vi "Range Kontrol X.vi"(0 "denge degeri":dbl, 1 "iterasyon Denge":dbl=1.0, 2 "frekans index":dbl, 3 "Denge Kosulu x1_x2":dbl[][](array[numeric]), 4 "Xk":dbl, 5 "X(k-1)":dbl=0.1, 6 "output x 1":dbl, 7 "output x 2":dbl) -> (14 "Output X(k-1)":dbl format="%.4p", 15 "result output x":dbl, 17 "KONTROL Y":bool, 18 "IF ELSE":bool, 19 "Start Denge Y":bool)   [LabVIEW 2014]
uses:
  Sub_VI/show_sensitivity.vi
  Sub_VI/global get findinput.vi
panel:
  in  "GPIB In":refnum<visa-resource-name>="GPIB0::8::INSTR"
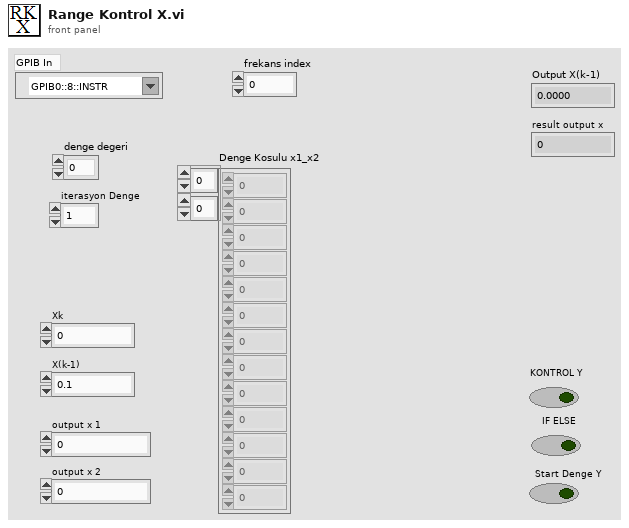
[diagram p1: front panel]
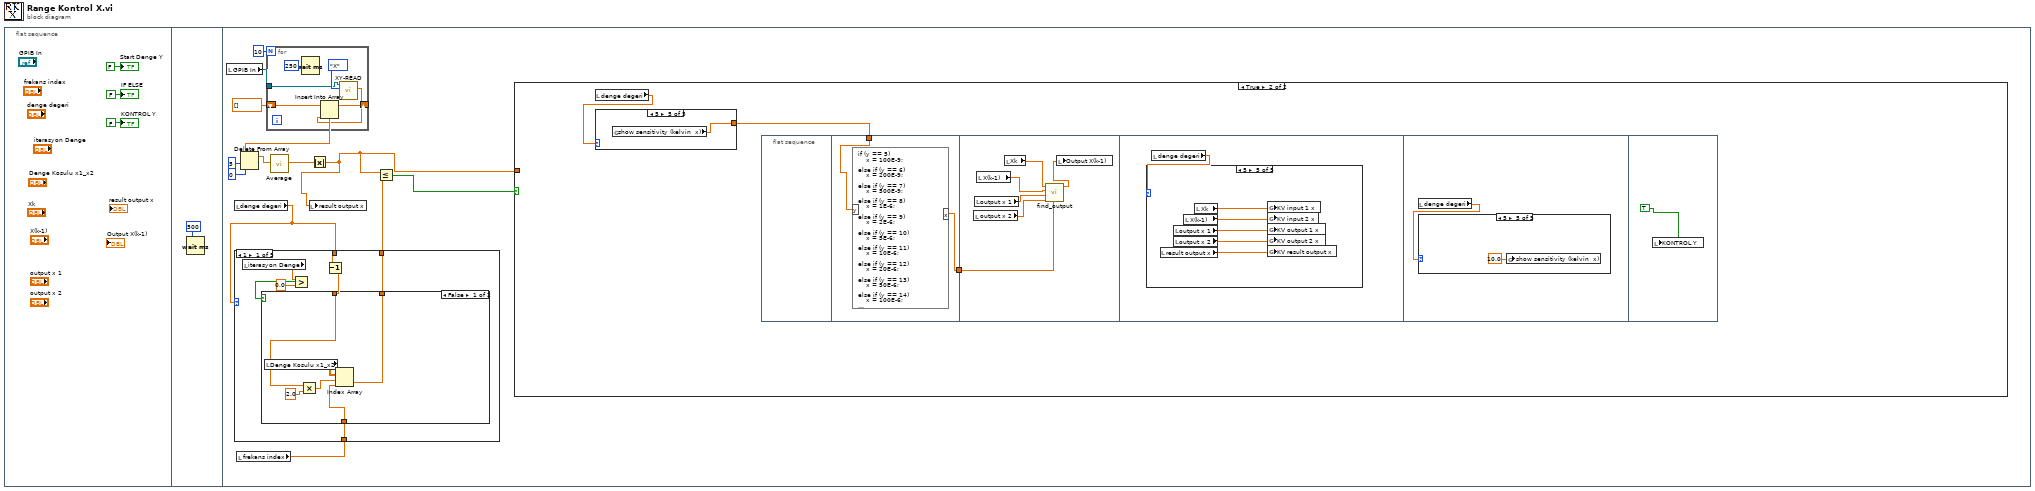
[diagram p0: block diagram]
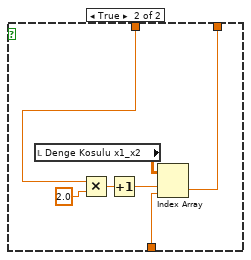
[diagram p2: hidden frame]
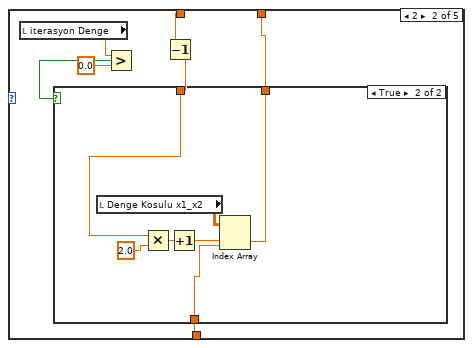
[diagram p3: hidden frame]
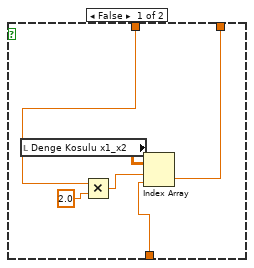
[diagram p4: hidden frame]
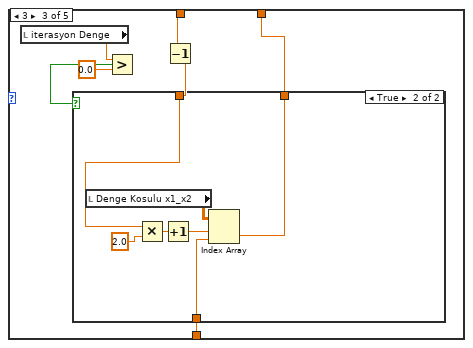
[diagram p5: hidden frame]
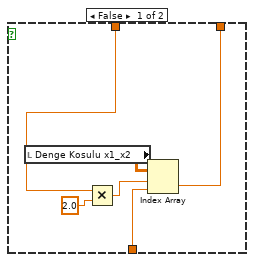
[diagram p6: hidden frame]
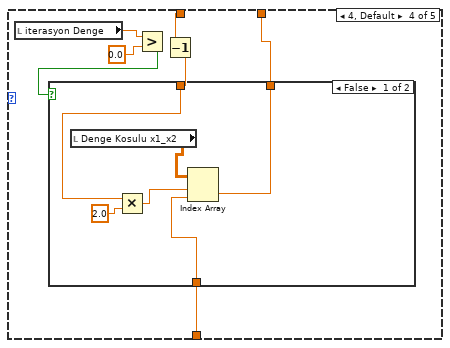
[diagram p7: hidden frame]
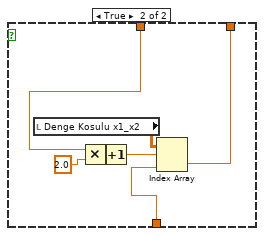
[diagram p8: hidden frame]
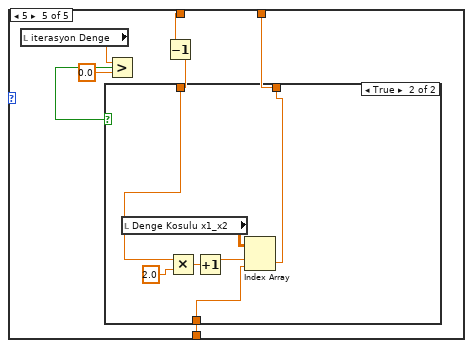
[diagram p9: hidden frame]
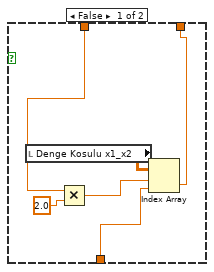
[diagram p10: hidden frame]
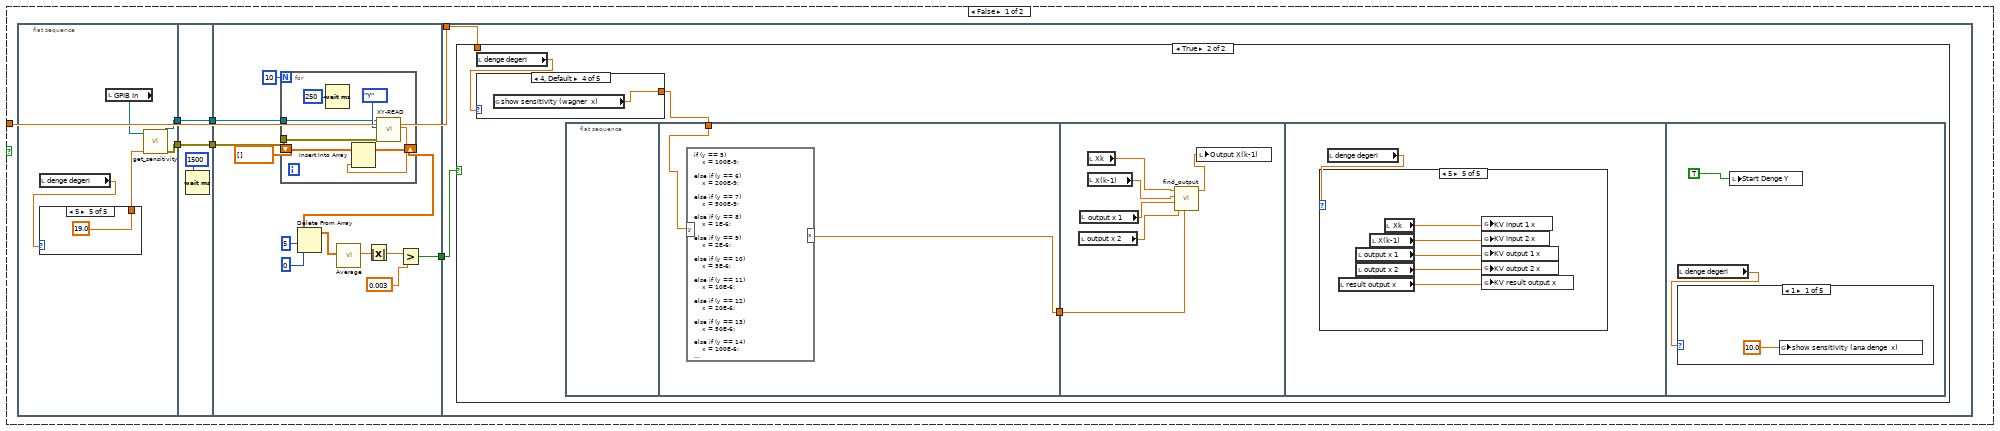
[diagram p11: hidden frame]
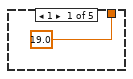
[diagram p12: hidden frame]
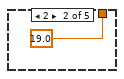
[diagram p13: hidden frame]
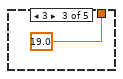
[diagram p14: hidden frame]
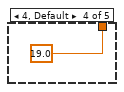
[diagram p15: hidden frame]
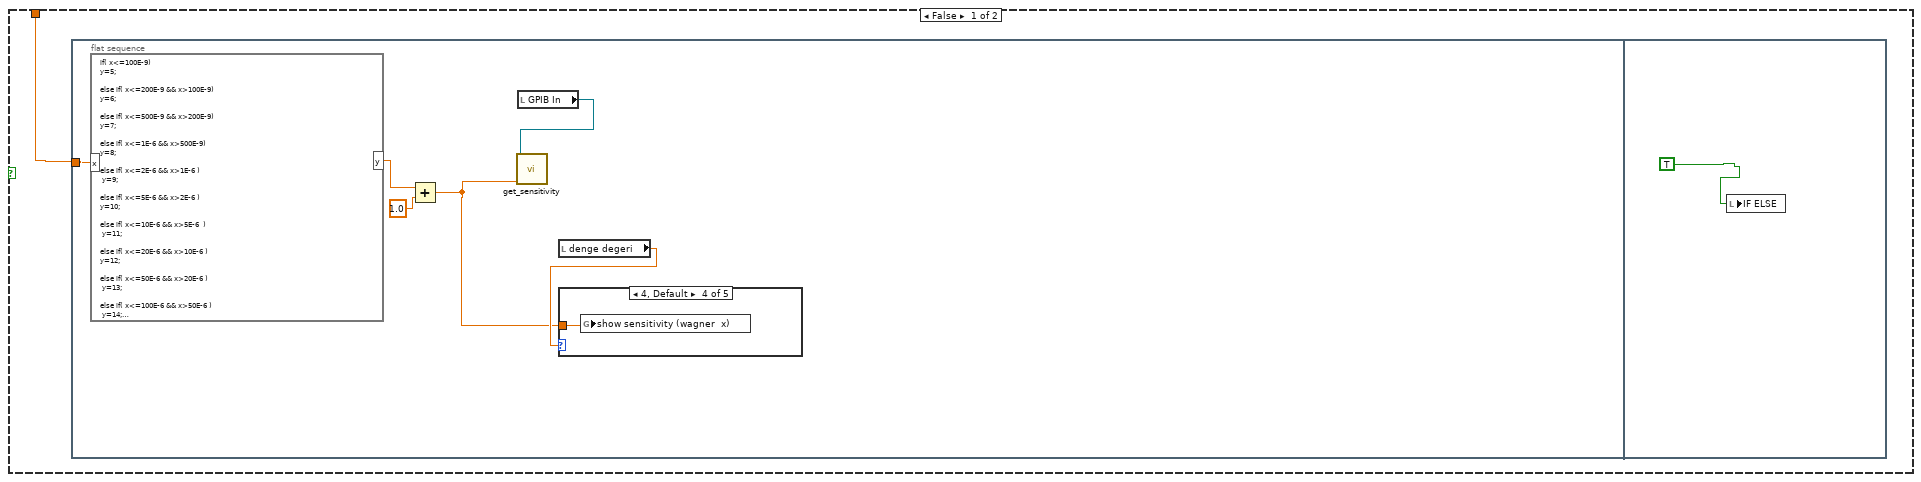
[diagram p16: hidden frame]
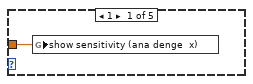
[diagram p17: hidden frame]
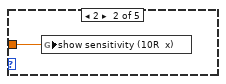
[diagram p18: hidden frame]
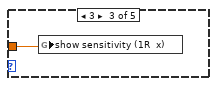
[diagram p19: hidden frame]
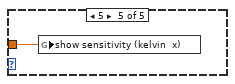
[diagram p20: hidden frame]
diagram:
  n1 = flat-sequence {
    frame #0 {
      "Start Denge Y" <- FALSE ("Denge Y")
      "IF ELSE" <- FALSE ("IF ELSE")
      "KONTROL Y" <- FALSE ("KONTROL Y")
    }
    frame #1 {
      n2 = Wait (ms)(milliseconds to wait=u32 500) -> ()  [unwired: 1 out]
    }
    frame #2 {
      n3 = local read "GPIB In"() -> (w5:refnum<visa-resource-name>)
      n4 = local read "denge degeri"() -> (w8:dbl)
      n5 = local read "frekans index"() -> (w6:dbl)
      n6 = case shown="1" w8 {
        tunnel: [w21 w41 w61 w84 w101] -> w9
        tunnel: w8 -> [w20 w40 w60 w80 w100]
        tunnel: w6 -> [w18 w38 w58 w78 w98]
        frame 1 {
          n7 = local read "iterasyon Denge"() -> (w23:dbl)
          n8 = Greater?(x=w23, y=0.0) -> (0:w24:bool)
          n9 = Decrement(x=w20) -> (x-1=w19:dbl)
          n10 = case shown="False" w24 {
            tunnel: [w28 w34] -> w21
            tunnel: w19 -> [w27 w33]
            tunnel: w18 -> [w25 w31]
            frame False {
              n11 = local read "Denge Kosulu x1_x2"() -> (w30:dbl[][])
              n12 = Multiply(x=w27, y=2.0) -> (x*y=w26:dbl)
              n13 = Index Array(array=w30, index (row)=w26, index (col)=w25) -> (element=w28:dbl)
            }
            frame True {
              n14 = local read "Denge Kosulu x1_x2"() -> (w35:dbl[][])
              n15 = Multiply(x=w33, y=2.0) -> (x*y=w37:dbl)
              n16 = Increment(x=w37) -> (x+1=w32:dbl)
              n17 = Index Array(array=w35, index (row)=w32, index (col)=w31) -> (element=w34:dbl)
            }
          }
        }
        frame 2 {
          n18 = local read "iterasyon Denge"() -> (w43:dbl)
          n19 = Greater?(x=w43, y=0.0) -> (0:w44:bool)
          n20 = Decrement(x=w40) -> (x-1=w39:dbl)
          n21 = case shown="True" w44 {
            tunnel: [w48 w54] -> w41
            tunnel: w39 -> [w47 w53]
            tunnel: w38 -> [w45 w51]
            frame False {
              n22 = local read "Denge Kosulu x1_x2"() -> (w50:dbl[][])
              n23 = Multiply(x=w47, y=2.0) -> (x*y=w46:dbl)
              n24 = Index Array(array=w50, index (row)=w46, index (col)=w45) -> (element=w48:dbl)
            }
            frame True {
              n25 = local read "Denge Kosulu x1_x2"() -> (w55:dbl[][])
              n26 = Multiply(x=w53, y=2.0) -> (x*y=w57:dbl)
              n27 = Increment(x=w57) -> (x+1=w52:dbl)
              n28 = Index Array(array=w55, index (row)=w52, index (col)=w51) -> (element=w54:dbl)
            }
          }
        }
        frame 3 {
          n29 = local read "iterasyon Denge"() -> (w62:dbl)
          n30 = Greater?(x=w62, y=0.0) -> (0:w64:bool)
          n31 = Decrement(x=w60) -> (x-1=w59:dbl)
          n32 = case shown="True" w64 {
            tunnel: [w68 w74] -> w61
            tunnel: w59 -> [w67 w73]
            tunnel: w58 -> [w65 w71]
            frame False {
              n33 = local read "Denge Kosulu x1_x2"() -> (w70:dbl[][])
              n34 = Multiply(x=w67, y=2.0) -> (x*y=w66:dbl)
              n35 = Index Array(array=w70, index (row)=w66, index (col)=w65) -> (element=w68:dbl)
            }
            frame True {
              n36 = local read "Denge Kosulu x1_x2"() -> (w75:dbl[][])
              n37 = Multiply(x=w73, y=2.0) -> (x*y=w77:dbl)
              n38 = Increment(x=w77) -> (x+1=w72:dbl)
              n39 = Index Array(array=w75, index (row)=w72, index (col)=w71) -> (element=w74:dbl)
            }
          }
        }
        frame 4, Default {
          n40 = local read "iterasyon Denge"() -> (w82:dbl)
          n41 = Greater?(x=w82, y=0.0) -> (0:w81:bool)
          n42 = Decrement(x=w80) -> (x-1=w79:dbl)
          n43 = case shown="False" w81 {
            tunnel: [w88 w94] -> w84
            tunnel: w79 -> [w87 w93]
            tunnel: w78 -> [w85 w91]
            frame False {
              n44 = local read "Denge Kosulu x1_x2"() -> (w90:dbl[][])
              n45 = Multiply(x=w87, y=2.0) -> (x*y=w86:dbl)
              n46 = Index Array(array=w90, index (row)=w86, index (col)=w85) -> (element=w88:dbl)
            }
            frame True {
              n47 = local read "Denge Kosulu x1_x2"() -> (w95:dbl[][])
              n48 = Multiply(x=w93, y=2.0) -> (x*y=w97:dbl)
              n49 = Increment(x=w97) -> (x+1=w92:dbl)
              n50 = Index Array(array=w95, index (row)=w92, index (col)=w91) -> (element=w94:dbl)
            }
          }
        }
        frame 5 {
          n51 = local read "iterasyon Denge"() -> (w102:dbl)
          n52 = Greater?(x=w102, y=0.0) -> (0:w104:bool)
          n53 = Decrement(x=w100) -> (x-1=w99:dbl)
          n54 = case shown="True" w104 {
            tunnel: [w108 w114] -> w101
            tunnel: w99 -> [w107 w113]
            tunnel: w98 -> [w105 w111]
            frame False {
              n55 = local read "Denge Kosulu x1_x2"() -> (w110:dbl[][])
              n56 = Multiply(x=w107, y=2.0) -> (x*y=w106:dbl)
              n57 = Index Array(array=w110, index (row)=w106, index (col)=w105) -> (element=w108:dbl)
            }
            frame True {
              n58 = local read "Denge Kosulu x1_x2"() -> (w115:dbl[][])
              n59 = Multiply(x=w113, y=2.0) -> (x*y=w117:dbl)
              n60 = Increment(x=w117) -> (x+1=w112:dbl)
              n61 = Index Array(array=w115, index (row)=w112, index (col)=w111) -> (element=w114:dbl)
            }
          }
        }
      }
      n62 = for {
        N: 10 -> [_]
        shift-right: [w271] -> w14
        shift-left: dbl[] [] -> [w272]
        tunnel: w5 -> [w269]
        n63 = Wait (ms)(milliseconds to wait=u32 250) -> ()  [unwired: 1 out]
        n64 = call "XY-READ.vi"("X/Y ?"=enum16{"X", "Y"}."X" ("Enum"), "SR850 GPIB IN"=w269) -> ("SR850_Reading"=w273:dbl)  [unwired: 7 in, 2 out]
        n65 = Insert Into Array(array=w272, new element=w273) -> (w271:dbl[])  [unwired: 1 in]
      }
      n66 = Delete From Array(array=w14, length=5, index=0) -> (array with subset deleted=w15:dbl[])  [unwired: 1 out]
      n67 = call "Average.vi"("Array"=w15) -> ("Average"=w11:dbl)  [unwired: 9 in, 1 out]
      n68 = Absolute Value(x=w11) -> (abs(x)=w7:dbl)
      n69 = local write "result output x"(w7) -> ()
      n70 = Less Or Equal?(x=w7, y=w9) -> (x <= y?=w10:bool)
      n71 = case shown="True" w10 {
        tunnel: w7 -> [w118 _]
        frame False {
          n72 = flat-sequence {
            tunnel: [w127] -> w122
            tunnel: [w126] -> w120
            tunnel: [w135] -> w123
            tunnel: w122 -> [w135]
            tunnel: [w134] -> w121
            tunnel: w120 -> [w134]
            tunnel: w123 -> [w142]
            tunnel: w121 -> [w141]
            tunnel: [w138] -> w119
            tunnel: w119 -> [w157]
            tunnel: w118 -> [w156]
            frame #0 {
              n73 = local read "denge degeri"() -> (w125:dbl)
              n74 = case shown="5" w125 {
                tunnel: [19.0 ("input 1") 19.0 ("input 1") 19.0 ("input 1") 19.0 ("input 1") 19.0 ("input 1")] -> w124
                frame 1 {
                }
                frame 2 {
                }
                frame 3 {
                }
                frame 4, Default {
                }
                frame 5 {
                }
              }
              n75 = local read "GPIB In"() -> (w128:refnum<visa-resource-name>)
              n76 = call "get_sensitivity.vi"("input 1"=w124, "SR850 GPIB In"=w128) -> ("error out"=w126:errorcluster, "SR850 GPIB Out"=w127:refnum<visa-resource-name>)  [unwired: 8 in]
            }
            frame #1 {
              n77 = Wait (ms)(milliseconds to wait=u32 1500) -> ()  [unwired: 1 out]
            }
            frame #2 {
              n78 = for {
                N: 10 -> [_]
                tunnel: w142 -> [w154]
                tunnel: w141 -> [w153]
                shift-right: [w150] -> w146
                shift-left: dbl[] [] -> [w151]
                n79 = Wait (ms)(milliseconds to wait=u32 250) -> ()  [unwired: 1 out]
                n80 = call "XY-READ.vi"("Error IN"=w153, "X/Y ?"=enum16{"X", "Y"}."Y" ("Enum"), "SR850 GPIB IN"=w154) -> ("SR850_Reading"=w152:dbl)  [unwired: 6 in, 2 out]
                n81 = Insert Into Array(array=w151, new element=w152) -> (w150:dbl[])  [unwired: 1 in]
              }
              n82 = Delete From Array(array=w146, length=5, index=0) -> (array with subset deleted=w145:dbl[])  [unwired: 1 out]
              n83 = call "Average.vi"("Array"=w145) -> ("Average"=w139:dbl)  [unwired: 9 in, 1 out]
              n84 = Absolute Value(x=w139) -> (abs(x)=w137:dbl)
              n85 = Greater?(x=w137, y=0.003) -> (0:w138:bool)
            }
            frame #3 {
              n86 = case shown="True" w157 {
                tunnel: w156 -> [w158 _]
                frame False {
                  n87 = flat-sequence {
                    tunnel: w158 -> [w163]
                    frame #0 {
                      n88 = formula code="if( x<=100E-9) \ny=5;\n\nelse if( x<=200E-9 && x>100E-9) \ny=6;\n\nelse if( x<=500E-9 && x>200E-9) \ny=7;\n\nelse if( x<=1E-6 && x>500E-9) \ny=8;\n\nelse if( x<=2E-6 && x>1E-6 ) \n\ty=9;\n\nelse if( x<=5E-6 && x>2E-6 ) \ny=10;\n\nelse if( x<=10E-6 && x>5E-6  ) \n\ty=11;\n\nelse if( x<=20E-6 && x>10E-6 ) \ny=12;\n\nelse if( x<=50E-6 && x>20E-6 ) \n\ty=13;\n\nelse if( x<=100E-6 && x>50E-6 ) \n\ty=14;\n\nelse if( x<=200E-6 && x>100E-6 ) \n\ty=15;\n\nelse if( x<=500E-6 && x>200E-6 ) \n\ty=16;\n\nelse if(  x<=1E-3 && x>500E-6 ) \n\ty=17;\n\nelse if( x<=2E-3 && x>1E-3 ) \n\ty=18;\n\nelse if(  x<=5E-3 && x>2E-3) \ny=19;\n\nelse if(  x<=10E-3 && x>5E-3 ) \n\ty=20;\n\nelse if(  x<=20E-3 && x>10E-3) \n\ty=21;\n\nelse if(  x<=50E-3 && x>20E-3 ) \n\ty=22;\n\nelse if(  x<=100E-3 && x>50E-3 ) \n\ty=23;\n\nelse if(  x<=200E-3 && x>100E-3 ) \n\ty=24;\n\nelse if(  x<=500E-3 && x>200E-3 ) \n\ty=25;\n\nelse if(  x<=1 && x>500E-3 ) \ny=26;\n\nelse \n\ty=26;"("x"=w163) -> ("y"=w161:dbl)
                      n89 = Add(x=w161, y=1.0) -> (x+y=w159:dbl)
                      n90 = local read "GPIB In"() -> (w164:refnum<visa-resource-name>)
                      n91 = call "get_sensitivity.vi"("input 1"=w159, "SR850 GPIB In"=w164) -> ()  [unwired: 8 in, 2 out]
                      n92 = local read "denge degeri"() -> (w162:dbl)
                      n93 = case shown="4, Default" w162 {
                        tunnel: w159 -> [w165 w166 w167 w168 w169]
                        frame 1 {
                          n94 = global write "show_sensitivity.vi" "show sensitivity (ana denge  x)"(w165) -> ()
                        }
                        frame 2 {
                          n95 = global write "show_sensitivity.vi" "show sensitivity (10R  x)"(w166) -> ()
                        }
                        frame 3 {
                          n96 = global write "show_sensitivity.vi" "show sensitivity (1R  x)"(w167) -> ()
                        }
                        frame 4, Default {
                          n97 = global write "show_sensitivity.vi" "show sensitivity (wagner  x)"(w168) -> ()
                        }
                        frame 5 {
                          n98 = global write "show_sensitivity.vi" "show sensitivity (kelvin  x)"(w169) -> ()
                        }
                      }
                    }
                    frame #1 {
                      n99 = local write "IF ELSE"(TRUE ("if else")) -> ()
                    }
                  }
                }
                frame True {
                  n100 = local read "denge degeri"() -> (w172:dbl)
                  n101 = case shown="4, Default" w172 {
                    tunnel: [w174 w175 w176 w177 w178] -> w171
                    frame 1 {
                      n102 = global read "show_sensitivity.vi" "show sensitivity (ana denge  x)"() -> (w174:dbl)
                    }
                    frame 2 {
                      n103 = global read "show_sensitivity.vi" "show sensitivity (10R  x)"() -> (w175:dbl)
                    }
                    frame 3 {
                      n104 = global read "show_sensitivity.vi" "show sensitivity (1R  x)"() -> (w176:dbl)
                    }
                    frame 4, Default {
                      n105 = global read "show_sensitivity.vi" "show sensitivity (wagner  x)"() -> (w177:dbl)
                    }
                    frame 5 {
                      n106 = global read "show_sensitivity.vi" "show sensitivity (kelvin  x)"() -> (w178:dbl)
                    }
                  }
                  n107 = flat-sequence {
                    tunnel: w171 -> [w179]
                    tunnel: [w180] -> w173
                    tunnel: w173 -> [w184]
                    frame #0 {
                    }
                    frame #1 {
                      n108 = formula code="if (y == 5) \n    x = 100E-9;\n\nelse if (y == 6) \n    x = 200E-9;\n\nelse if (y == 7) \n    x = 500E-9;\n\nelse if (y == 8) \n    x = 1E-6;\n\nelse if (y == 9) \n    x = 2E-6;\n\nelse if (y == 10) \n    x = 5E-6;\n\nelse if (y == 11) \n    x = 10E-6;\n\nelse if (y == 12) \n    x = 20E-6;\n\nelse if (y == 13) \n    x = 50E-6;\n\nelse if (y == 14) \n    x = 100E-6;\n\nelse if (y == 15) \n    x = 200E-6;\n\nelse if (y == 16) \n    x = 500E-6;\n\nelse if (y == 17) \n    x = 1E-3;\n\nelse if (y == 18) \n    x = 2E-3;\n\nelse if (y == 19) \n    x = 5E-3;\n\nelse if (y == 20) \n    x = 10E-3;\n\nelse if (y == 21) \n    x = 20E-3;\n\nelse if (y == 22) \n    x = 50E-3;\n\nelse if (y == 23) \n    x = 100E-3;\n\nelse if (y == 24) \n    x = 200E-3;\n\nelse if (y == 25) \n    x = 500E-3;\n\nelse if (y == 26) \n    x = 1;\n\nelse \n    x = 1;"("y"=w179) -> ("x"=w180:dbl)
                    }
                    frame #2 {
                      n109 = local read "output x 2"() -> (w185:dbl)
                      n110 = local read "output x 1"() -> (w186:dbl)
                      n111 = local read "Xk"() -> (w181:dbl)
                      n112 = local read "X(k-1)"() -> (w182:dbl)
                      n113 = call "find_output.vi"("find output"=w184, "output 2"=w185, "output 1"=w186, "input 2"=w182, "input 1"=w181) -> ("getInput"=w183:dbl)  [unwired: 6 in]
                      n114 = local write "Output X(k-1)"(w183) -> ()
                    }
                    frame #3 {
                      n115 = local read "denge degeri"() -> (w187:dbl)
                      n116 = case shown="5" w187 {
                        frame 1 {
                          n117 = local read "result output x"() -> (w188:dbl)
                          n118 = local read "output x 1"() -> (w190:dbl)
                          n119 = local read "output x 2"() -> (w189:dbl)
                          n120 = local read "X(k-1)"() -> (w191:dbl)
                          n121 = local read "Xk"() -> (w192:dbl)
                          n122 = global write "global get findinput.vi" "AD input 1 x"(w192) -> ()
                          n123 = global write "global get findinput.vi" "AD input 2 x"(w191) -> ()
                          n124 = global write "global get findinput.vi" "AD output 1 x"(w190) -> ()
                          n125 = global write "global get findinput.vi" "AD output 2 x"(w189) -> ()
                          n126 = global write "global get findinput.vi" "AD result output x"(w188) -> ()
                        }
                        frame 2 {
                          n127 = local read "result output x"() -> (w193:dbl)
                          n128 = local read "output x 1"() -> (w195:dbl)
                          n129 = local read "output x 2"() -> (w194:dbl)
                          n130 = local read "X(k-1)"() -> (w196:dbl)
                          n131 = local read "Xk"() -> (w197:dbl)
                          n132 = global write "global get findinput.vi" "10R input 1 x"(w197) -> ()
                          n133 = global write "global get findinput.vi" "10R input 2 x"(w196) -> ()
                          n134 = global write "global get findinput.vi" "10R output 1 x"(w195) -> ()
                          n135 = global write "global get findinput.vi" "10R output 2 x"(w194) -> ()
                          n136 = global write "global get findinput.vi" "10R result output x"(w193) -> ()
                        }
                        frame 3 {
                          n137 = local read "result output x"() -> (w198:dbl)
                          n138 = local read "output x 1"() -> (w200:dbl)
                          n139 = local read "output x 2"() -> (w199:dbl)
                          n140 = local read "X(k-1)"() -> (w201:dbl)
                          n141 = local read "Xk"() -> (w202:dbl)
                          n142 = global write "global get findinput.vi" "1R input 1 x"(w202) -> ()
                          n143 = global write "global get findinput.vi" "1R input 2 x"(w201) -> ()
                          n144 = global write "global get findinput.vi" "1R output 1 x"(w200) -> ()
                          n145 = global write "global get findinput.vi" "1R output 2 x"(w199) -> ()
                          n146 = global write "global get findinput.vi" "1R result output x"(w198) -> ()
                        }
                        frame 4, Default {
                          n147 = local read "result output x"() -> (w203:dbl)
                          n148 = local read "output x 1"() -> (w205:dbl)
                          n149 = local read "output x 2"() -> (w204:dbl)
                          n150 = local read "X(k-1)"() -> (w206:dbl)
                          n151 = local read "Xk"() -> (w207:dbl)
                          n152 = global write "global get findinput.vi" "W input 1 x"(w207) -> ()
                          n153 = global write "global get findinput.vi" "W input 2 x"(w206) -> ()
                          n154 = global write "global get findinput.vi" "W output 1 x"(w205) -> ()
                          n155 = global write "global get findinput.vi" "W output 2 x"(w204) -> ()
                          n156 = global write "global get findinput.vi" "W result output x"(w203) -> ()
                        }
                        frame 5 {
                          n157 = local read "result output x"() -> (w208:dbl)
                          n158 = local read "output x 1"() -> (w209:dbl)
                          n159 = local read "output x 2"() -> (w210:dbl)
                          n160 = local read "X(k-1)"() -> (w211:dbl)
                          n161 = local read "Xk"() -> (w212:dbl)
                          n162 = global write "global get findinput.vi" "KV input 1 x"(w212) -> ()
                          n163 = global write "global get findinput.vi" "KV input 2 x"(w211) -> ()
                          n164 = global write "global get findinput.vi" "KV output 1 x"(w209) -> ()
                          n165 = global write "global get findinput.vi" "KV output 2 x"(w210) -> ()
                          n166 = global write "global get findinput.vi" "KV result output x"(w208) -> ()
                        }
                      }
                    }
                    frame #4 {
                      n167 = local read "denge degeri"() -> (w213:dbl)
                      n168 = case shown="1" w213 {
                        frame 1 {
                          n169 = global write "show_sensitivity.vi" "show sensitivity (ana denge  x)"(10.0 ("show sensitivity (kelvin  x)")) -> ()
                        }
                        frame 2 {
                          n170 = global write "show_sensitivity.vi" "show sensitivity (10R  x)"(16.0 ("show sensitivity (kelvin  x)")) -> ()
                        }
                        frame 3 {
                          n171 = global write "show_sensitivity.vi" "show sensitivity (1R  x)"(16.0 ("show sensitivity (kelvin  x)")) -> ()
                        }
                        frame 4, Default {
                          n172 = global write "show_sensitivity.vi" "show sensitivity (wagner  x)"(16.0 ("show sensitivity (kelvin  x)")) -> ()
                        }
                        frame 5 {
                          n173 = global write "show_sensitivity.vi" "show sensitivity (kelvin  x)"(10.0 ("show sensitivity (kelvin  x)")) -> ()
                        }
                      }
                      n174 = local write "Start Denge Y"(TRUE ("WAGNER Y")) -> ()
                    }
                  }
                }
              }
            }
          }
        }
        frame True {
          n175 = local read "denge degeri"() -> (w222:dbl)
          n176 = case shown="5" w222 {
            tunnel: [w264 w265 w266 w267 w268] -> w220
            frame 1 {
              n177 = global read "show_sensitivity.vi" "show sensitivity (ana denge  x)"() -> (w264:dbl)
            }
            frame 2 {
              n178 = global read "show_sensitivity.vi" "show sensitivity (10R  x)"() -> (w265:dbl)
            }
            frame 3 {
              n179 = global read "show_sensitivity.vi" "show sensitivity (1R  x)"() -> (w266:dbl)
            }
            frame 4, Default {
              n180 = global read "show_sensitivity.vi" "show sensitivity (wagner  x)"() -> (w267:dbl)
            }
            frame 5 {
              n181 = global read "show_sensitivity.vi" "show sensitivity (kelvin  x)"() -> (w268:dbl)
            }
          }
          n182 = flat-sequence {
            tunnel: w220 -> [w223]
            tunnel: [w224] -> w221
            tunnel: w221 -> [w228]
            frame #0 {
            }
            frame #1 {
              n183 = formula code="if (y == 5) \n    x = 100E-9;\n\nelse if (y == 6) \n    x = 200E-9;\n\nelse if (y == 7) \n    x = 500E-9;\n\nelse if (y == 8) \n    x = 1E-6;\n\nelse if (y == 9) \n    x = 2E-6;\n\nelse if (y == 10) \n    x = 5E-6;\n\nelse if (y == 11) \n    x = 10E-6;\n\nelse if (y == 12) \n    x = 20E-6;\n\nelse if (y == 13) \n    x = 50E-6;\n\nelse if (y == 14) \n    x = 100E-6;\n\nelse if (y == 15) \n    x = 200E-6;\n\nelse if (y == 16) \n    x = 500E-6;\n\nelse if (y == 17) \n    x = 1E-3;\n\nelse if (y == 18) \n    x = 2E-3;\n\nelse if (y == 19) \n    x = 5E-3;\n\nelse if (y == 20) \n    x = 10E-3;\n\nelse if (y == 21) \n    x = 20E-3;\n\nelse if (y == 22) \n    x = 50E-3;\n\nelse if (y == 23) \n    x = 100E-3;\n\nelse if (y == 24) \n    x = 200E-3;\n\nelse if (y == 25) \n    x = 500E-3;\n\nelse if (y == 26) \n    x = 1;\n\nelse \n    x = 1;"("y"=w223) -> ("x"=w224:dbl)
            }
            frame #2 {
              n184 = local read "output x 2"() -> (w229:dbl)
              n185 = local read "output x 1"() -> (w230:dbl)
              n186 = local read "X(k-1)"() -> (w226:dbl)
              n187 = local read "Xk"() -> (w225:dbl)
              n188 = call "find_output.vi"("find output"=w228, "output 2"=w229, "output 1"=w230, "input 2"=w226, "input 1"=w225) -> ("getInput"=w227:dbl)  [unwired: 6 in]
              n189 = local write "Output X(k-1)"(w227) -> ()
            }
            frame #3 {
              n190 = local read "denge degeri"() -> (w231:dbl)
              n191 = case shown="5" w231 {
                frame 1 {
                  n192 = local read "result output x"() -> (w232:dbl)
                  n193 = local read "output x 1"() -> (w234:dbl)
                  n194 = local read "output x 2"() -> (w233:dbl)
                  n195 = local read "X(k-1)"() -> (w235:dbl)
                  n196 = local read "Xk"() -> (w236:dbl)
                  n197 = global write "global get findinput.vi" "AD input 1 x"(w236) -> ()
                  n198 = global write "global get findinput.vi" "AD input 2 x"(w235) -> ()
                  n199 = global write "global get findinput.vi" "AD output 1 x"(w234) -> ()
                  n200 = global write "global get findinput.vi" "AD output 2 x"(w233) -> ()
                  n201 = global write "global get findinput.vi" "AD result output x"(w232) -> ()
                }
                frame 2 {
                  n202 = local read "result output x"() -> (w237:dbl)
                  n203 = local read "output x 1"() -> (w239:dbl)
                  n204 = local read "output x 2"() -> (w238:dbl)
                  n205 = local read "X(k-1)"() -> (w240:dbl)
                  n206 = local read "Xk"() -> (w241:dbl)
                  n207 = global write "global get findinput.vi" "10R input 1 x"(w241) -> ()
                  n208 = global write "global get findinput.vi" "10R input 2 x"(w240) -> ()
                  n209 = global write "global get findinput.vi" "10R output 1 x"(w239) -> ()
                  n210 = global write "global get findinput.vi" "10R output 2 x"(w238) -> ()
                  n211 = global write "global get findinput.vi" "10R result output x"(w237) -> ()
                }
                frame 3 {
                  n212 = local read "result output x"() -> (w242:dbl)
                  n213 = local read "output x 1"() -> (w244:dbl)
                  n214 = local read "output x 2"() -> (w243:dbl)
                  n215 = local read "X(k-1)"() -> (w245:dbl)
                  n216 = local read "Xk"() -> (w246:dbl)
                  n217 = global write "global get findinput.vi" "1R input 1 x"(w246) -> ()
                  n218 = global write "global get findinput.vi" "1R input 2 x"(w245) -> ()
                  n219 = global write "global get findinput.vi" "1R output 1 x"(w244) -> ()
                  n220 = global write "global get findinput.vi" "1R output 2 x"(w243) -> ()
                  n221 = global write "global get findinput.vi" "1R result output x"(w242) -> ()
                }
                frame 4, Default {
                  n222 = local read "result output x"() -> (w247:dbl)
                  n223 = local read "output x 1"() -> (w249:dbl)
                  n224 = local read "output x 2"() -> (w248:dbl)
                  n225 = local read "X(k-1)"() -> (w250:dbl)
                  n226 = local read "Xk"() -> (w251:dbl)
                  n227 = global write "global get findinput.vi" "W input 1 x"(w251) -> ()
                  n228 = global write "global get findinput.vi" "W input 2 x"(w250) -> ()
                  n229 = global write "global get findinput.vi" "W output 1 x"(w249) -> ()
                  n230 = global write "global get findinput.vi" "W output 2 x"(w248) -> ()
                  n231 = global write "global get findinput.vi" "W result output x"(w247) -> ()
                }
                frame 5 {
                  n232 = local read "result output x"() -> (w252:dbl)
                  n233 = local read "output x 1"() -> (w253:dbl)
                  n234 = local read "output x 2"() -> (w254:dbl)
                  n235 = local read "X(k-1)"() -> (w255:dbl)
                  n236 = local read "Xk"() -> (w256:dbl)
                  n237 = global write "global get findinput.vi" "KV input 1 x"(w256) -> ()
                  n238 = global write "global get findinput.vi" "KV input 2 x"(w255) -> ()
                  n239 = global write "global get findinput.vi" "KV output 1 x"(w253) -> ()
                  n240 = global write "global get findinput.vi" "KV output 2 x"(w254) -> ()
                  n241 = global write "global get findinput.vi" "KV result output x"(w252) -> ()
                }
              }
            }
            frame #4 {
              n242 = local read "denge degeri"() -> (w257:dbl)
              n243 = case shown="5" w257 {
                frame 1 {
                  n244 = global write "show_sensitivity.vi" "show sensitivity (ana denge  x)"(10.0 ("show sensitivity (kelvin  x)")) -> ()
                }
                frame 2 {
                  n245 = global write "show_sensitivity.vi" "show sensitivity (10R  x)"(16.0 ("show sensitivity (kelvin  x)")) -> ()
                }
                frame 3 {
                  n246 = global write "show_sensitivity.vi" "show sensitivity (1R  x)"(16.0 ("show sensitivity (kelvin  x)")) -> ()
                }
                frame 4, Default {
                  n247 = global write "show_sensitivity.vi" "show sensitivity (wagner  x)"(16.0 ("show sensitivity (kelvin  x)")) -> ()
                }
                frame 5 {
                  n248 = global write "show_sensitivity.vi" "show sensitivity (kelvin  x)"(10.0 ("show sensitivity (kelvin  x)")) -> ()
                }
              }
            }
            frame #5 {
              n249 = local write "KONTROL Y"(TRUE ("KONTROL Y")) -> ()
            }
          }
        }
      }
    }
  }
